vi "LENGTH OF FIRST NAME AND LAST NAME.vi"() -> ()   [LabVIEW 2015]
panel:
  out "substring":string
  in  "Table":string[][](table)
  out "SIZE OF FIRST NAME":i32
  out "SIZE OF SECOND NAME":i32
  out "SECOND NAME":string
  out "FIRST NAME":string
  in  "STING ARRAY":string[](array[string])
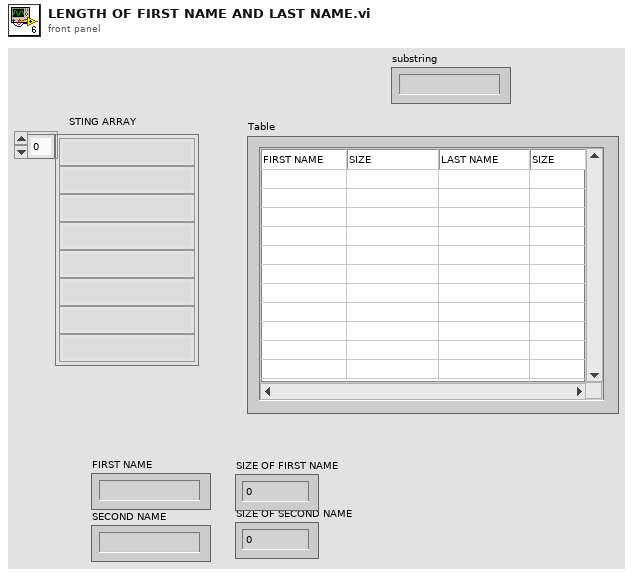
[diagram p1: front panel]
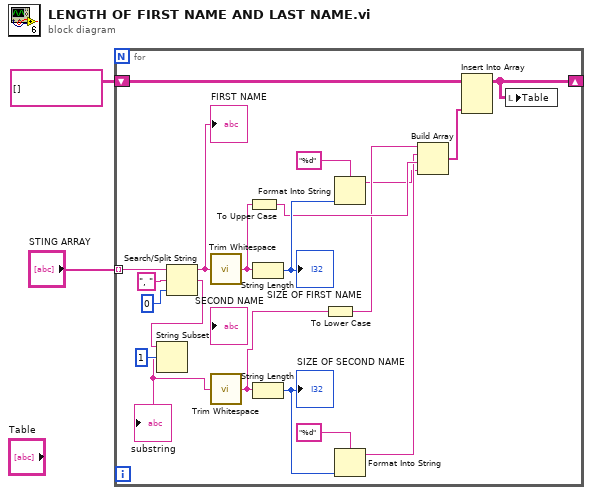
[diagram p0: block diagram]
diagram:
  n1 = for {
    tunnel: "STING ARRAY" -> [w22] mode=indexing
    shift-right: [w18] -> _
    shift-left: string[][] [] -> [w19]
    n2 = Search/Split String(string=w22, search string/char (-)=", ", offset (0)=0) -> (substring before match=w17:string, match + rest of string=w3:string)  [unwired: 1 out]
    "FIRST NAME" <- w17
    n3 = String Subset(string=w3, offset (0)=1) -> (substring=w4:string)  [unwired: 1 in]
    "substring" <- w4
    n4 = call <vilib>:"Trim Whitespace.vi"("string"=w17) -> ("trimmed string"=w11:string)  [unwired: 1 in]
    n5 = call <vilib>:"Trim Whitespace.vi"("string"=w4) -> ("trimmed string"=w9:string)  [unwired: 1 in]
    n6 = To Upper Case(1:w11) -> (0:w10:string)
    n7 = String Length(string=w11) -> (length=w16:i32)
    "SIZE OF FIRST NAME" <- w16
    n8 = String Length(string=w9) -> (length=w14:i32)
    "SIZE OF SECOND NAME" <- w14
    n9 = To Lower Case(string=w9) -> (all lower case string=w8:string)
    n10 = Format Into String(format string="%d", w16) -> (resulting string=w6:string)  [unwired: 2 in, 1 out]
    n11 = Format Into String(format string="%d", w14) -> (resulting string=w7:string)  [unwired: 2 in, 1 out]
    n12 = Build Array(w8, w7, w10, w6) -> (w12:string[])
    n13 = Insert Into Array(array=w19, new element=w12) -> (w18:string[][])  [unwired: 2 in]
    n14 = local write "Table"(w18) -> ()
  }
